vi "RobotDriveMecanumDrive_Custom.vi"(6 "Rotation":dbl, 7 "Gyro Angle":dbl, 8 "error in (no error)":errorcluster, 9 "Y":dbl, 10 "X":dbl, 11 "RobotDriveDevRef":T1={"DevStatus"={"status"=FALSE, "code"=0, "source"=""}, "Motors[]"=[], "Square Inputs"=FALSE, "Max Output"=1.0}) -> (0 "error out":errorcluster, 2 "Motor Values":dbl[](array[numeric]), 3 "RobotDriveDevRef":T1={"DevStatus"={"status"=FALSE, "code"=0, "source"=""}, "Motors[]"=[], "Square Inputs"=FALSE, "Max Output"=1.0})   [LabVIEW 2014]
doc: "Configures the motors for holonomic driving. Holonomic driving allows you to move the robot in any direction without first rotating or maneuvering the robot.\n\nThis VI requires the robot to have either four omni-directional wheels and four motors mounted at 45 degree angles in the four corners of a square frame or to have four mecanum wheels driven by four motors.\n\nThe control input is intended to be connected directly to the X, Y, and Z axes of a joystick. The Y axis is inverted for you.\n\nThis software is licensed. Open the labview\\readme\\WPI Robotics Library Open Source License.txt file for more information."
uses:
  <vilib>/Rock Robotics/WPI/RobotDrive/WPI_RobotDriveDevRef.ctl
  <vilib>/Rock Robotics/WPI/MotorControl/WPI_MotorControlDeviceRef.ctl
  <vilib>/Rock Robotics/WPI/MotorControl/WPI_MotorControlType.ctl
  <vilib>/Rock Robotics/SystemInterfaces/Typedef/FPGA_TypedefDigitalModule.ctl
  <vilib>/Rock Robotics/SystemInterfaces/DIO/FPGA_DIOPWMChannel.ctl
  <vilib>/Rock Robotics/WPI/PWM/WPI_PWMDeadband.ctl
  <vilib>/Rock Robotics/WPI/CAN/Jaguar/SubVIs/WPI_CANJaguar_ControlMode.ctl
  <vilib>/Rock Robotics/WPI/CAN/TalonSRX/WPI_CANTalonSRX_APIControlMode.ctl
  <vilib>/Rock Robotics/WPI/PWM/WPI_PWMTransform_ConPane.ctl
  <vilib>/Rock Robotics/SystemInterfaces/NetworkCommunication/NetComm_UsageReport_ResourceType.ctl
  <vilib>/Rock Robotics/WPI/RobotDrive/WPI_RobotDriveMotorSelectorEnum.ctl
  Robot Global Data.vi
  <vilib>/Rock Robotics/WPI/RobotDrive/WPI_RobotDriveSafetyCheck.vi
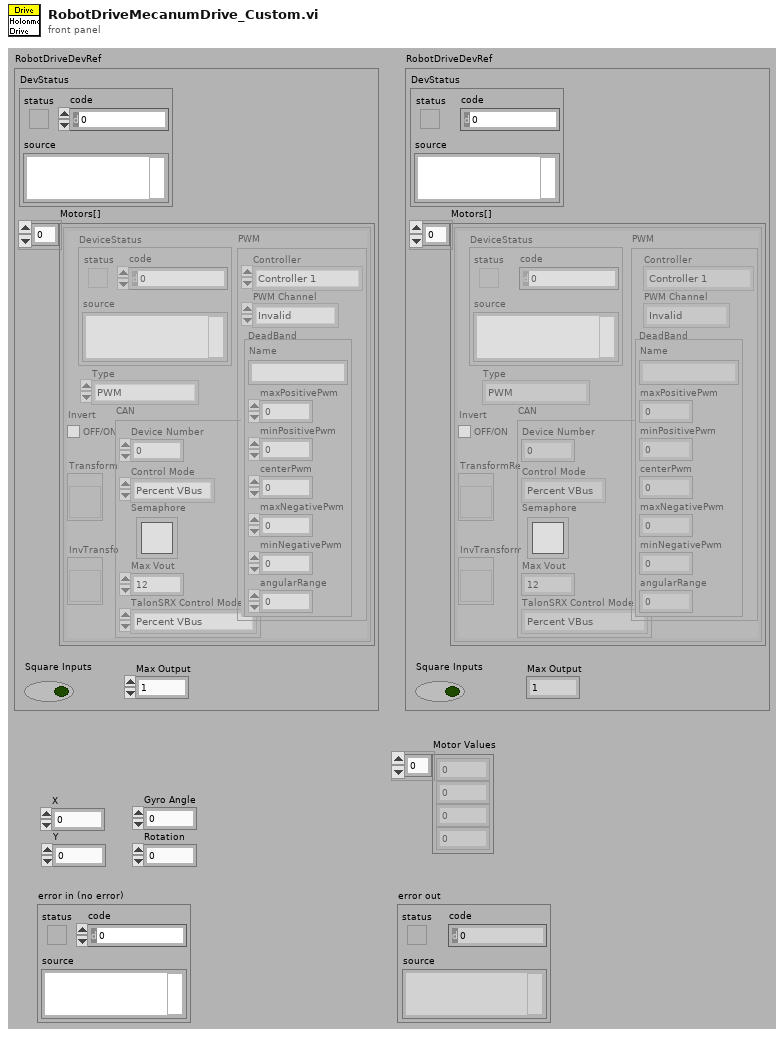
[diagram p1: front panel]
types:
  T1 = typedef "WPI_RobotDriveDevRef.ctl" = cluster{"DevStatus":errorcluster, "Motors[]":T2[], "Square Inputs":bool, "Max Output":dbl}
  T2 = typedef "WPI_MotorControlDeviceRef.ctl" = cluster{"DeviceStatus":errorcluster, "Type":T3, "PWM":cluster{"Controller":T4, "PWM Channel":T5, "DeadBand":T6}, "CAN":cluster{"Device Number":u8, "Control Mode":T7, "Semaphore":T8, "Max Vout":dbl, "TalonSRX Control Mode":T9}, "Invert":bool, "TransformRef":T10, "InvTransformRef":T10}
  T3 = typedef "WPI_MotorControlType.ctl" = enum16{"PWM", "CAN", "CANTalonSRX"}
  T4 = typedef "FPGA_TypedefDigitalModule.ctl" = enum16{"Controller 1"}
  T5 = typedef "FPGA_DIOPWMChannel.ctl" = enum8{"PWM 0", "PWM 1", "PWM 2", "PWM 3", "PWM 4", "PWM 5", "PWM 6", "PWM 7", "PWM 8", "PWM 9", "PWM MXP 0", "PWM MXP 1", "PWM MXP 2", "PWM MXP 3", "PWM MXP 4", "PWM MXP 5", "PWM MXP 6", "PWM MXP 7", "PWM MXP 8", "PWM MXP 9", "Invalid"}
  T6 = typedef "WPI_PWMDeadband.ctl" = cluster{"Name":string, "maxPositivePwm":i32, "minPositivePwm":i32, "centerPwm":i32, "maxNegativePwm":i32, "minNegativePwm":i32, "angularRange":u16}
  T7 = typedef "WPI_CANJaguar_ControlMode.ctl" = enum8{"Percent VBus", "Current", "Speed", "Position", "Voltage"}
  T8 = typedef "Semaphore RefNum" = refnum<k1>
  T9 = typedef "WPI_CANTalonSRX_APIControlMode.ctl" = enum8{"Percent VBus", "Speed", "Position", "Slave", "Unchanged / Invalid"}
  T10 = typedef "WPI_PWMTransform_ConPane.ctl" = refnum<vi>
  T11 = typedef "NetComm_UsageReport_ResourceType.ctl" = enum8{"Controller", "Module", "Language", "CANPlugin", "Accelerometer", "ADXL345", "AnalogChannel", "AnalogTrigger", "AnalogTriggerOutput", "CANJaguar", "Compressor", "Counter", "Dashboard", "DigitalInput", "DigitalOutput", "DriverStationCIO", "DriverStationEIO", "DriverStationLCD", "Encoder", "GearTooth", "Gyro", "I2C", "Framework", "Jaguar", "Joystick", "Kinect", "KinectStick", "PIDController", "Preferences", "PWM", "Relay", "RobotDrive", "SerialPort", "Servo", "Solenoid", "SPI", "Task", "Ultrasonic", "Victor", "Button", "Command", "AxisCamera", "PCVideoServer", "SmartDashboard", "Talon", "HiTechnicColorSensor", "HiTechnicAccel", "HiTechnicCompass", "SRF08", "AnalogOutput", "Victor SP", "Talon SRX", "CAN Talon SRX"}
  T12 = typedef "WPI_RobotDriveMotorSelectorEnum.ctl" = enum16{"Rear Left Motor", "Rear Right Motor", "Front Left Motor", "Front Right Motor"}
  T13 = typedef "WPI_CANTalonSRX_GlobalStatus.ctl" = cluster{"Applied Throttle":dbl, "Module Enabled":bool, "CAN Error":errorcluster, "Closed Loop Error":dbl, "Forward Limit Switch Closed":bool, "Reverse Limit Switch Closed":bool, "Sensor Position":dbl, "Sensor Velocity":dbl, "Current":dbl, "Sticky Fault - Over Temp":bool, "Sticky Fault - Under Voltage":bool, "Sticky Fault - Forward Limit":bool, "Sticky Fault - Reverse Limit":bool, "Sticky Fault - Forward Soft Limit":bool, "Sticky Fault - Reverse Soft Limit":bool, "Brake is Enabled":bool, "Encoder Position":dbl, "Encoder Velocity":dbl, "Encoder Index Count":dbl, "Encoder A Pin State":bool, "Encoder B Pin State":bool, "Encoder Index Pin State":bool, "Analog In":dbl, "Analog In Velocity":dbl, "Temperature (C)":dbl, "Battery Voltage":dbl}
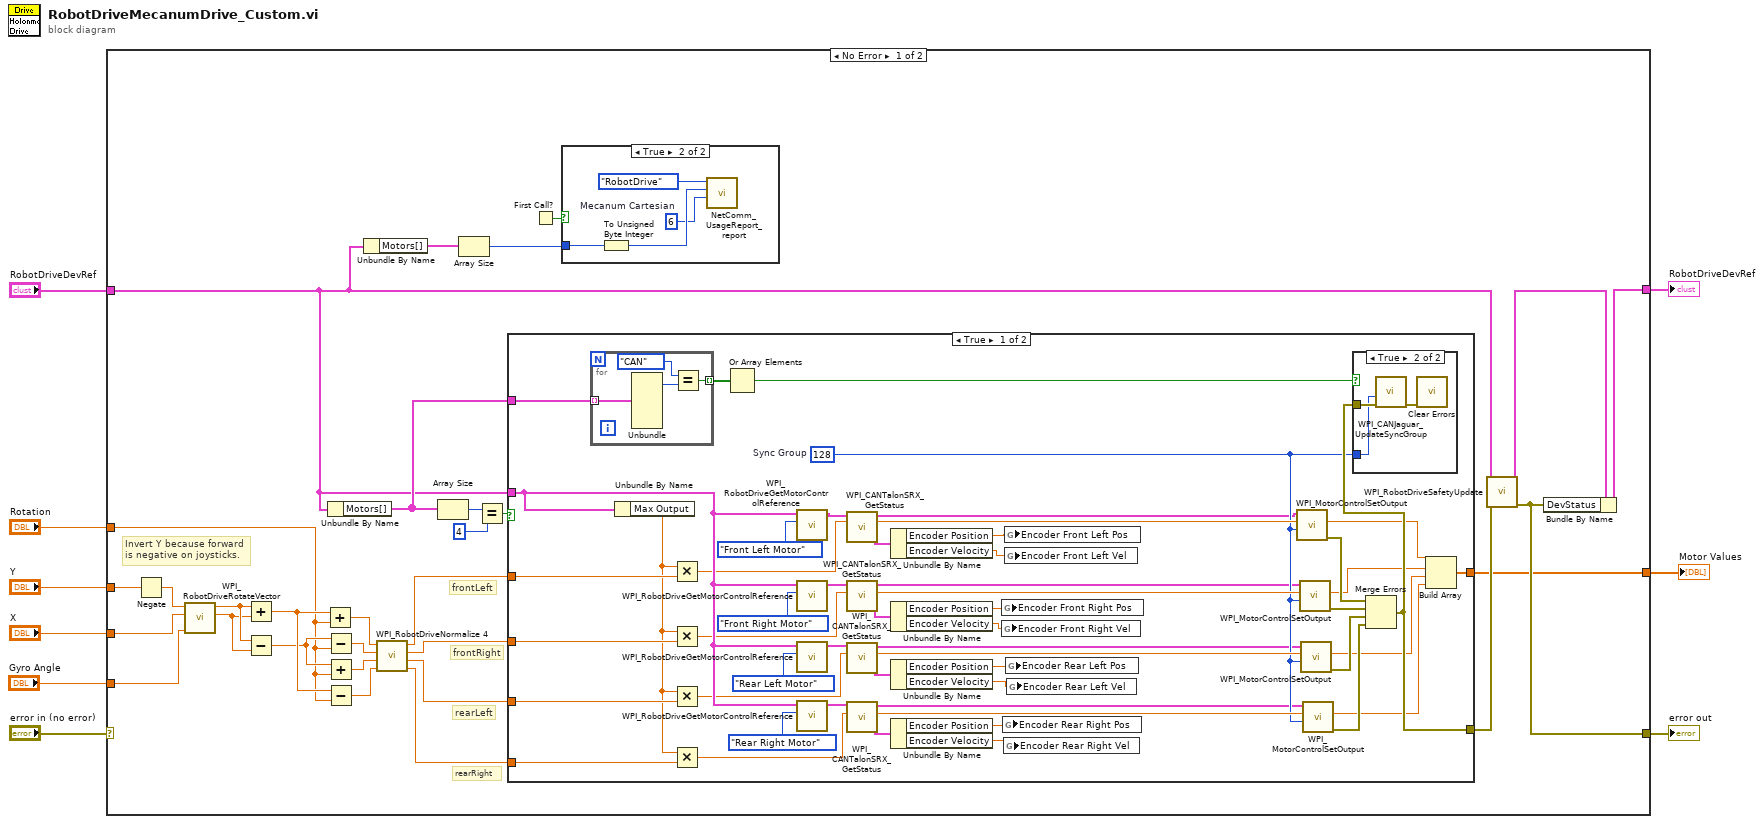
[diagram p0: block diagram]
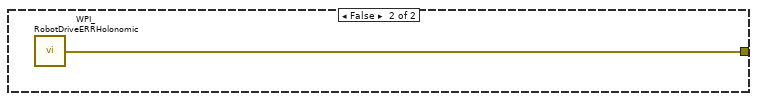
[diagram p4: hidden frame]
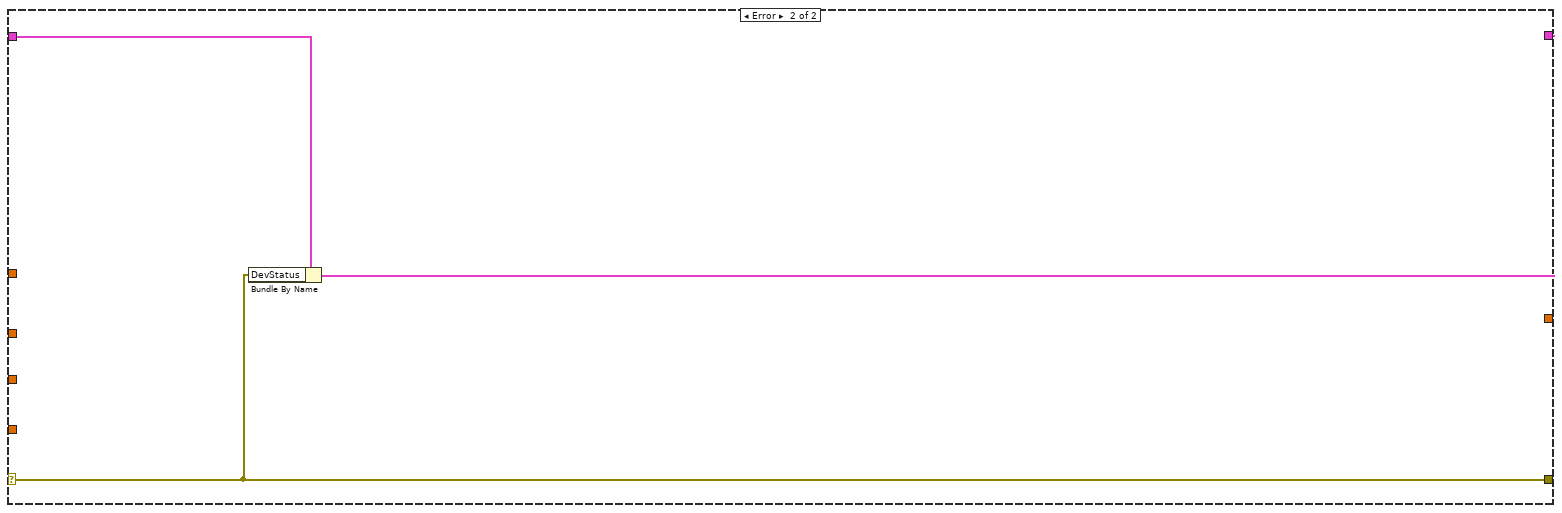
[diagram p5: hidden frame]
diagram:
  n1 = case shown="No Error" "error in (no error)" {
    selector: "error in (no error)" -> [_ w100]
    tunnel: "Y" -> [w21 _]
    tunnel: "X" -> [w26 _]
    tunnel: "RobotDriveDevRef" -> [w11 w102]
    tunnel: [w36 w101] -> w5
    tunnel: [w16 w100] -> w4
    tunnel: "Rotation" -> [w27 _]
    tunnel: "Gyro Angle" -> [w20 _]
    tunnel: [w10 _] -> w1
    frame No Error {
      # "Invert Y because forward is negative on joysticks."
      # "rearLeft"
      # "frontRight"
      # "rearRight"
      # "frontLeft"
      n2 = Negate(x=w21) -> (-x=w19:dbl)
      n3 = call <vilib>:"WPI_RobotDriveRotateVector.vi"("Angle"=w20, "X"=w26, "Y"=w19) -> ("X'"=w34:dbl, "Y'"=w35:dbl)  [unwired: 7 out]
      n4 = Add(x=w35, y=w34) -> (x+y=w32:dbl)
      n5 = Subtract(x=w35, y=w34) -> (x-y=w30:dbl)
      n6 = Add(x=w32, y=w27) -> (x+y=w28:dbl)
      n7 = Subtract(x=w30, y=w27) -> (x-y=w29:dbl)
      n8 = Add(x=w30, y=w27) -> (x+y=w31:dbl)
      n9 = Subtract(x=w32, y=w27) -> (x-y=w33:dbl)
      n10 = Unbundle By Name(w11) -> ("Motors[]"=w15:T2[])
      n11 = Unbundle By Name(w11) -> ("Motors[]"=w13:T2[])
      n12 = call <vilib>:"WPI_RobotDriveNormalize 4.vi"("D"=w33, "C"=w31, "B"=w29, "A"=w28) -> ("D'"=w23:dbl, "C'"=w22:dbl, "B'"=w24:dbl, "A'"=w25:dbl)
      n13 = Array Size(array=w15) -> (size(s)=w39:i32)
      n14 = Array Size(array=w13) -> (size(s)=w12:i32)
      n15 = Equal?(x=w39, y=4) -> (x = y?=w37:bool)
      n16 = case shown="True" w37 {
        tunnel: w25 -> [w91 _]
        tunnel: w24 -> [w90 _]
        tunnel: w11 -> [w83 _]
        tunnel: [w70 w99] -> w18
        tunnel: w22 -> [w89 _]
        tunnel: w23 -> [w88 _]
        tunnel: w15 -> [w71 _]
        tunnel: [w67 _] -> w10
        frame True {
          w69 = u8 128  # Sync Group
          n17 = for {
            tunnel: w71 -> [w95] mode=indexing
            tunnel: [w92] -> w72 mode=indexing
            n18 = Unbundle(w95) -> ("Type"=w94:T3)  [unwired: 6 out]
            n19 = Equal?(x=enum16{"PWM", "CAN"}."CAN" ("Type"), y=w94) -> (x = y?=w92:bool)
          }
          n20 = Unbundle By Name(w83) -> ("Max Output"=w78:dbl)
          n21 = Multiply(x=w78, y=w91) -> (x*y=w82:dbl)
          n22 = Multiply(x=w78, y=w90) -> (x*y=w81:dbl)
          n23 = Multiply(x=w78, y=w89) -> (x*y=w80:dbl)
          n24 = Multiply(x=w78, y=w88) -> (x*y=w79:dbl)
          n25 = Or Array Elements(Boolean array=w72) -> (logical OR=w73:bool)
          n26 = call <vilib>:"WPI_RobotDriveGetMotorControlReference.vi"("MotorIndex"=WPI_RobotDriveMotorSelectorEnum."Front Left Motor", "RobotDriveDevRef"=w83) -> ("MotorControlDeviceRef"=w63:T2)  [unwired: 9 out]
          n27 = call <vilib>:"WPI_RobotDriveGetMotorControlReference.vi"("MotorIndex"=WPI_RobotDriveMotorSelectorEnum."Front Right Motor", "RobotDriveDevRef"=w83) -> ("MotorControlDeviceRef"=w55:T2)  [unwired: 9 out]
          n28 = call <vilib>:"WPI_RobotDriveGetMotorControlReference.vi"("MotorIndex"=WPI_RobotDriveMotorSelectorEnum."Rear Left Motor", "RobotDriveDevRef"=w83) -> ("MotorControlDeviceRef"=w51:T2)  [unwired: 9 out]
          n29 = call <vilib>:"WPI_RobotDriveGetMotorControlReference.vi"("MotorIndex"=WPI_RobotDriveMotorSelectorEnum."Rear Right Motor", "RobotDriveDevRef"=w83) -> ("MotorControlDeviceRef"=w47:T2)  [unwired: 9 out]
          n30 = call <vilib>:"WPI_CANTalonSRX_GetStatus.vi"("CAN Talon SRX Ref"=w63) -> ("Talon SRX Status"=w61:T13, "CAN Talon SRX Ref Out"=w62:T2)  [unwired: 8 in, 1 out]
          n31 = call <vilib>:"WPI_CANTalonSRX_GetStatus.vi"("CAN Talon SRX Ref"=w55) -> ("Talon SRX Status"=w56:T13, "CAN Talon SRX Ref Out"=w46:T2)  [unwired: 8 in, 1 out]
          n32 = call <vilib>:"WPI_CANTalonSRX_GetStatus.vi"("CAN Talon SRX Ref"=w51) -> ("Talon SRX Status"=w54:T13, "CAN Talon SRX Ref Out"=w45:T2)  [unwired: 8 in, 1 out]
          n33 = call <vilib>:"WPI_CANTalonSRX_GetStatus.vi"("CAN Talon SRX Ref"=w47) -> ("Talon SRX Status"=w48:T13, "CAN Talon SRX Ref Out"=w44:T2)  [unwired: 8 in, 1 out]
          n34 = Unbundle By Name(w61) -> ("Encoder Position"=w59:dbl, "Encoder Velocity"=w60:dbl)
          n35 = Unbundle By Name(w56) -> ("Encoder Position"=w58:dbl, "Encoder Velocity"=w57:dbl)
          n36 = Unbundle By Name(w54) -> ("Encoder Position"=w52:dbl, "Encoder Velocity"=w53:dbl)
          n37 = Unbundle By Name(w48) -> ("Encoder Position"=w50:dbl, "Encoder Velocity"=w49:dbl)
          n38 = global write "Robot Global Data.vi" "Encoder Front Right Pos"(w58) -> ()
          n39 = global write "Robot Global Data.vi" "Encoder Front Right Vel"(w57) -> ()
          n40 = global write "Robot Global Data.vi" "Encoder Rear Right Pos"(w50) -> ()
          n41 = global write "Robot Global Data.vi" "Encoder Rear Right Vel"(w49) -> ()
          n42 = global write "Robot Global Data.vi" "Encoder Front Left Pos"(w59) -> ()
          n43 = global write "Robot Global Data.vi" "Encoder Front Left Vel"(w60) -> ()
          n44 = global write "Robot Global Data.vi" "Encoder Rear Left Pos"(w52) -> ()
          n45 = global write "Robot Global Data.vi" "Encoder Rear Left Vel"(w53) -> ()
          n46 = call <vilib>:"WPI_MotorControlSetOutput.vi"("Sync Group / Parameter Slot"=w69, "Output"=w82, "MotorControlDevRef"=w62) -> ("error out"=w74:errorcluster, "Motor Output"=w68:dbl)  [unwired: 2 in, 5 out]
          n47 = call <vilib>:"WPI_MotorControlSetOutput.vi"("Sync Group / Parameter Slot"=w69, "Output"=w81, "MotorControlDevRef"=w46) -> ("error out"=w75:errorcluster, "Motor Output"=w66:dbl)  [unwired: 2 in, 5 out]
          n48 = call <vilib>:"WPI_MotorControlSetOutput.vi"("Sync Group / Parameter Slot"=w69, "Output"=w80, "MotorControlDevRef"=w45) -> ("error out"=w76:errorcluster, "Motor Output"=w65:dbl)  [unwired: 2 in, 5 out]
          n49 = call <vilib>:"WPI_MotorControlSetOutput.vi"("Sync Group / Parameter Slot"=w69, "Output"=w79, "MotorControlDevRef"=w44) -> ("error out"=w77:errorcluster, "Motor Output"=w64:dbl)  [unwired: 2 in, 5 out]
          n50 = Merge Errors(w74, w75, w76, w77) -> (w70:errorcluster)
          n51 = case shown="True" w73 {
            tunnel: w70 -> [_ w97]
            tunnel: w69 -> [_ w96]
            frame False {
            }
            frame True {
              n52 = call <vilib>:"WPI_CANJaguar_UpdateSyncGroup.vi"("error in (no error)"=w97, "Sync Group"=w96) -> ("error out"=w98:errorcluster)  [unwired: 9 out]
              n53 = call <vilib>:"Clear Errors.vi"("error in (no error)"=w98) -> ()  [unwired: 1 in, 6 out]
            }
          }
          n54 = Build Array(w68, w66, w65, w64) -> (w67:dbl[])
        }
        frame False {
          n55 = call <vilib>:"WPI_RobotDriveERRHolonomic.vi"() -> ("error out"=w99:errorcluster)
        }
      }
      n56 = First Call?() -> (First Call?: T/F=w14:bool)
      n57 = case shown="True" w14 {
        tunnel: w12 -> [_ w42]
        frame False {
        }
        frame True {
          w40 = u8 6  # Mecanum Cartesian
          n58 = To Unsigned Byte Integer(number=w42) -> (unsigned 8bit integer=w41:u8)
          n59 = call <vilib>:"NetComm_UsageReport_report.vi"("Context"=w40, "Instance Number"=w41, "Resource Type"=NetComm_UsageReport_ResourceType."RobotDrive") -> ()  [unwired: 9 in]
        }
      }
      n60 = call <vilib>:"WPI_RobotDriveSafetyUpdate.vi"("error in (no error)"=w18, "RobotDriveDevRef"=w11) -> ("error out"=w16:errorcluster, "RobotDriveDevRef"=w17:T1)  [unwired: 8 out]
      n61 = Bundle By Name(cluster=w17, "DevStatus"=w16) -> (w36:T1)
    }
    frame Error {
      n62 = Bundle By Name(cluster=w102, "DevStatus"=w100) -> (w101:T1)
    }
  }
  "error out" <- w4
  "RobotDriveDevRef" <- w5
  "Motor Values" <- w1
